vi "BoxBoolean.vi"(10 "Boolean":bool) -> (2 "Boolean out":refnum<class "Boolean.lvclass">)   [LabVIEW 2013, in "LapDog.Collections.v1.Common.lvlib" / "Boolean.lvclass"]
uses:
  Boolean.lvclass
  Boolean.lvclass/Boolean.ctl
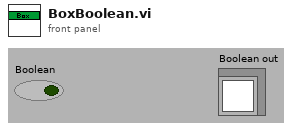
[diagram p1: front panel]
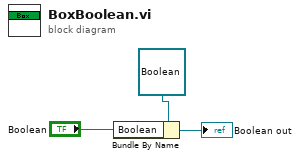
[diagram p0: block diagram]
diagram:
  n1 = Bundle By Name(cluster=refnum<class "Boolean.lvclass"> refnum ("LapDog.Collections.v0.Lists.Interfaces.lvlib:String.lvclass"), "Boolean"="Boolean") -> (→"Boolean out":refnum<class "Boolean.lvclass">)
